vi "GetVIPath(VIOrEXE).vi"(8 "error in (no error)":errorcluster, 11 "VI Name to Find":string) -> (0 "error out":errorcluster, 2 "VI or executable installation directory":path, 3 "Full Path to VI or executable":path)   [LabVIEW 2017, in "Client.lvlib"]
doc: "Current VI's Path (VI or exe).vi\n\n<B>Description:</B>\n\nThe Current VI's Path (VI or exe) VI is a drop-in replacement for the native Current VI's Path function. Just replace the native Current VI's Path function in your application with the Current VI's Path (VI or exe) VI and you'll never have to deal with the frustration caused by bad paths again -- whether you run your code in the development environment or as an executable!\n\nThe Current VI's Path (VI or exe) VI gets the path to the VI that called it and searches that path for \".exe\". If \".exe\" is found in the path, then the Current VI's Path (VI or exe) VI strips the path twice to obtain the executable's installation directory. If \".exe\" is not found, then the Current VI's Path (VI or exe) VI strips the path once to obtain the VI's installation directory.\n\nIn either case, the Current VI's Path (VI or exe) VI returns the VI or executable installation directory and the Full Path to the VI or executable. You can use this information in your application to easily access sub folders of the VI's or executable's installation directory by using the Build Path function to append the sub directory's name to the VI's or executable's installation path returned by the Current VI's Path (VI or exe) VI.\n\n<B>Usage:</B>\n\nUse the Current VI's Path (VI or exe) VI wherever you would use the native Current VI's Path function.\n\n<B>NOTES:</B>\n\nNone.\n\n<B>Inputs:</B>\n\nNone.\n\n<B>Outputs:</B>\n\nFull Path to VI or executable - The full path to the VI or executable.\n\nVI or executable installation directory - The path to the installation directory of the VI or executable.\n\n<B>Developed by:</B>\n\nMark Ridgley\nmark.ridgley@logicpd.com"
uses:
  <vilib>/Utility/error.llb/Error Cluster From Error Code.vi
  <vilib>/ErrorRing/Error Ring.xnode
  Client.lvlib
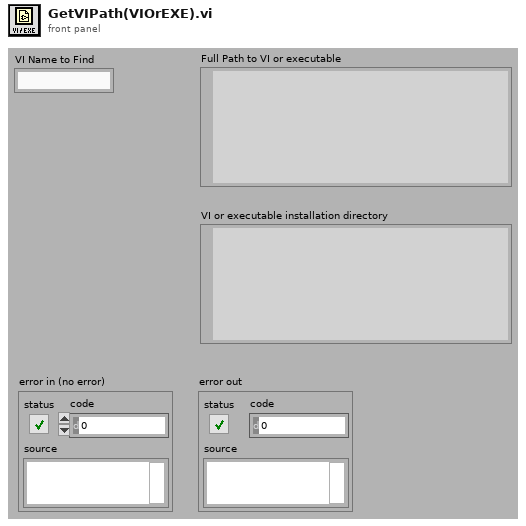
[diagram p1: front panel]
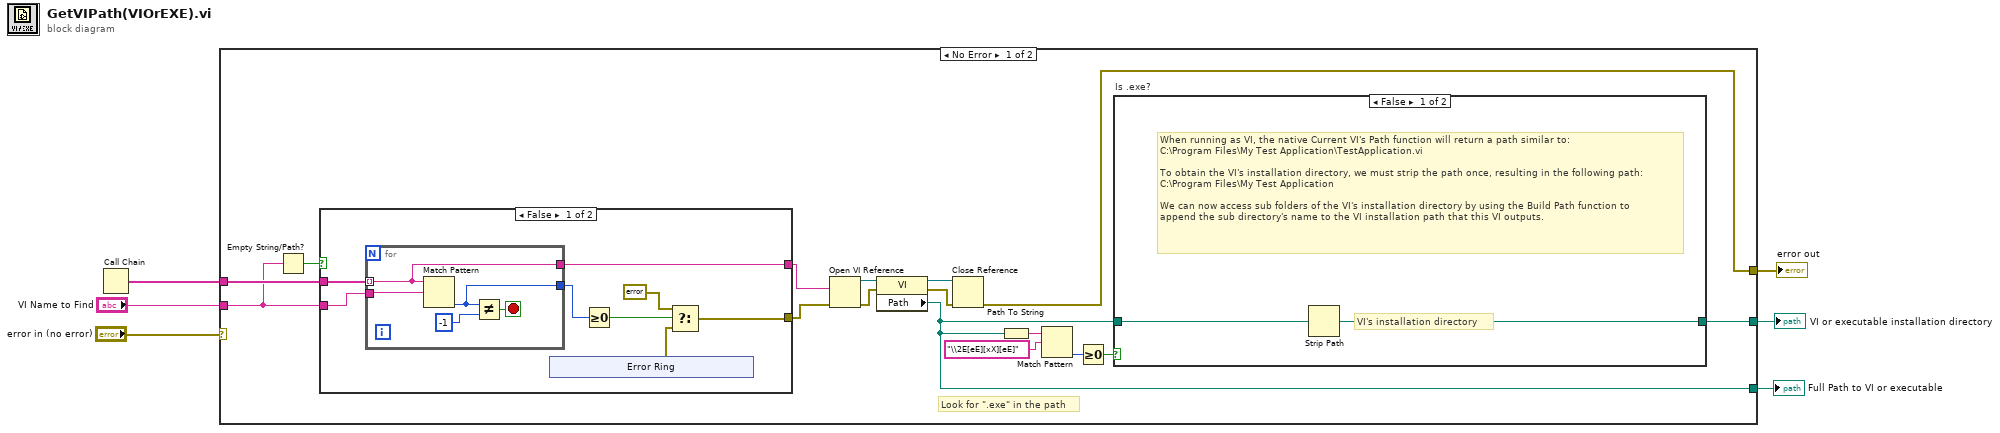
[diagram p0: block diagram]
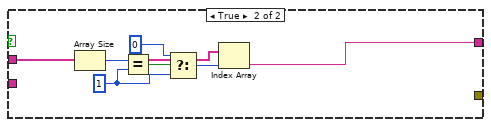
[diagram p2: hidden frame]
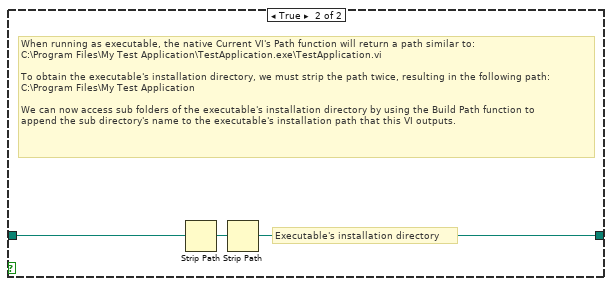
[diagram p3: hidden frame]
diagram:
  n1 = Call Chain() -> (call chain=w4:string[])
  n2 = case shown="No Error" "error in (no error)" {
    selector: "error in (no error)" -> [_ w53]
    tunnel: [w22 _] -> w6
    tunnel: [w14 _] -> w5
    tunnel: w4 -> [w11 _]
    tunnel: "VI Name to Find" -> [w9 _]
    tunnel: [w7 w53] -> w1
    frame No Error {
      # "Look for \".exe\" in the path"
      n3 = Empty String/Path?(string/path=w9) -> (empty?=w10:bool)
      n4 = case shown="False" w10 {
        tunnel: [w28 w42] -> w15
        tunnel: w11 -> [w29 w41]
        tunnel: w9 -> [w30 _]
        tunnel: [w23 _] -> w8
        frame False {
          n5 = for {
            tunnel: w29 -> [w37] mode=indexing
            tunnel: w30 -> [w40]
            tunnel: [w37] -> w28
            tunnel: [w36] -> w27
            stop <- w38 stop-if-true
            n6 = Match Pattern(string=w37, regular expression=w40) -> (offset past match=w36:i32)  [unwired: 1 in, 3 out]
            n7 = Not Equal?(x=w36, y=-1) -> (x != y?=w38:bool)
          }
          n8 = xnode "Error Ring"() -> ("error out"=w24:errorcluster)
          n9 = Greater Or Equal To 0?(x=w27) -> (x >= 0?=w26:bool)
          n10 = Select(t=errorcluster {"status"=FALSE, "code"=0, "source"=""} ("error in (no error)"), s=w26, f=w24) -> (s? t:f=w23:errorcluster)
        }
        frame True {
          w44 = 1 ("index")
          n11 = Array Size(array=w41) -> (size(s)=w45:i32)
          n12 = Equal?(x=w45, y=w44) -> (x = y?=w47:bool)
          n13 = Select(t=0, s=w47, f=w44) -> (s? t:f=w46:i32)
          n14 = Index Array(array=w41, index=w46) -> (element=w42:string)
        }
      }
      n15 = Open VI Reference(vi path=w15, error in (no error)=w8) -> (vi reference=w16:refnum<vi>, error out=w17:errorcluster)  [unwired: 4 in]
      n16 = property class="VI"(reference=w16, error in=w17) -> (reference out=w12:refnum<vi>, error out=w13:errorcluster, "Path"=w14:path)
      n17 = Close Reference(reference=w12, error in (no error)=w13) -> (error out=w7:errorcluster)
      n18 = Path To String(path=w14) -> (string=w19:string)
      n19 = Match Pattern(string=w19, regular expression="\\2E[eE][xX][eE]") -> (offset past match=w21:i32)  [unwired: 1 in, 3 out]
      n20 = Greater Or Equal To 0?(x=w21) -> (x >= 0?=w20:bool)
      n21 = case "Is .exe?" shown="False" w20 {
        tunnel: w14 -> [w49 w52]
        tunnel: [w48 w50] -> w22
        frame False {
          # "VI's installation directory"
          # "When running as VI, the native Current VI's Path function will return a path similar to:\nC:\\Program Files\\My Test Application\\TestApplication.vi\n\nTo obtain the VI's installation directory, we must strip the path once, resulting in the following path:\nC:\\Program Files\\My Test Application\n\nWe can now access sub folders of the VI's installation directory by using the Build Path function to\nappend the sub directory's name to the VI installation path that this VI outputs."
          n22 = Strip Path(path=w49) -> (stripped path=w48:path)  [unwired: 1 out]
        }
        frame True {
          # "Executable's installation directory"
          # "When running as executable, the native Current VI's Path function will return a path similar to:\nC:\\Program Files\\My Test Application\\TestApplication.exe\\TestApplication.vi\n\nTo obtain the executable's installation directory, we must strip the path twice, resulting in the following path:\nC:\\Program Files\\My Test Application\n\nWe can now access sub folders of the executable's installation directory by using the Build Path function to\nappend the sub directory's name to the executable's installation path that this VI outputs."
          n23 = Strip Path(path=w52) -> (stripped path=w51:path)  [unwired: 1 out]
          n24 = Strip Path(path=w51) -> (stripped path=w50:path)  [unwired: 1 out]
        }
      }
    }
    frame Error {
    }
  }
  "Full Path to VI or executable" <- w5
  "VI or executable installation directory" <- w6
  "error out" <- w1
